vi "Voltage to illuminance.vi"(8 "error in (no error)":errorcluster, 11 "Input Voltage (V)":dbl) -> (0 "error out":errorcluster, 3 "Illuminance (lx)":dbl)   [LabVIEW 2013]
doc: "Converts the input voltage to illuminance result."
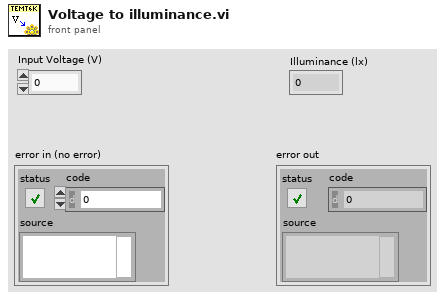
[diagram p1: front panel]
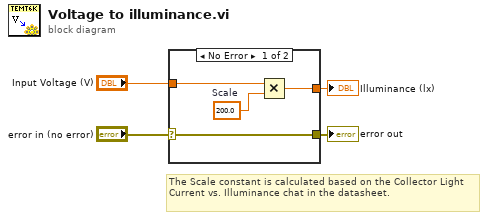
[diagram p0: block diagram]
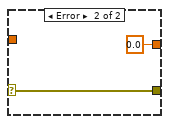
[diagram p2: hidden frame]
diagram:
  # "The Scale constant is calculated based on the Collector Light Current vs. Illuminance chat in the datasheet."
  n1 = case shown="No Error" "error in (no error)" {
    selector: "error in (no error)" -> [w5 w10]
    tunnel: "Input Voltage (V)" -> [w8 _]
    tunnel: [w6 0.0] -> w3
    tunnel: [w5 w10] -> w1
    frame No Error {
      w7 = 200.0  # Scale
      n2 = Multiply(x=w8, y=w7) -> (x*y=w6:dbl)
    }
    frame Error {
    }
  }
  "error out" <- w1
  "Illuminance (lx)" <- w3
